vi "Compute n x n Kernel (SGL).vi"(9 "Kernel Type":T1, 11 "Kernel Size":i32) -> (3 "Kernel":sgl[][](array[numeric]))   [LabVIEW 2021, in "Arrays.lvlib"]
uses:
  Arrays.lvlib
  Kernel Type.ctl
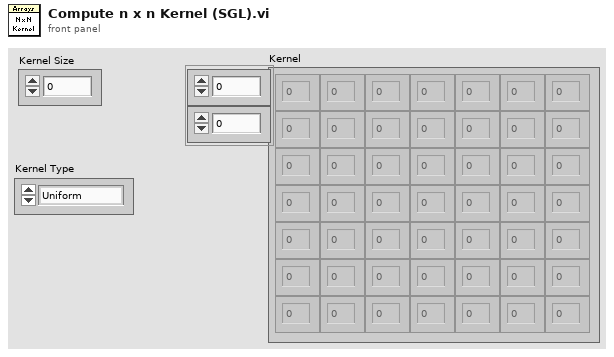
[diagram p1: front panel]
types:
  T1 = typedef "Arrays.lvlib/Kernel Type.ctl" = enum16{"Uniform", "Bilinear", "Gaussian"}
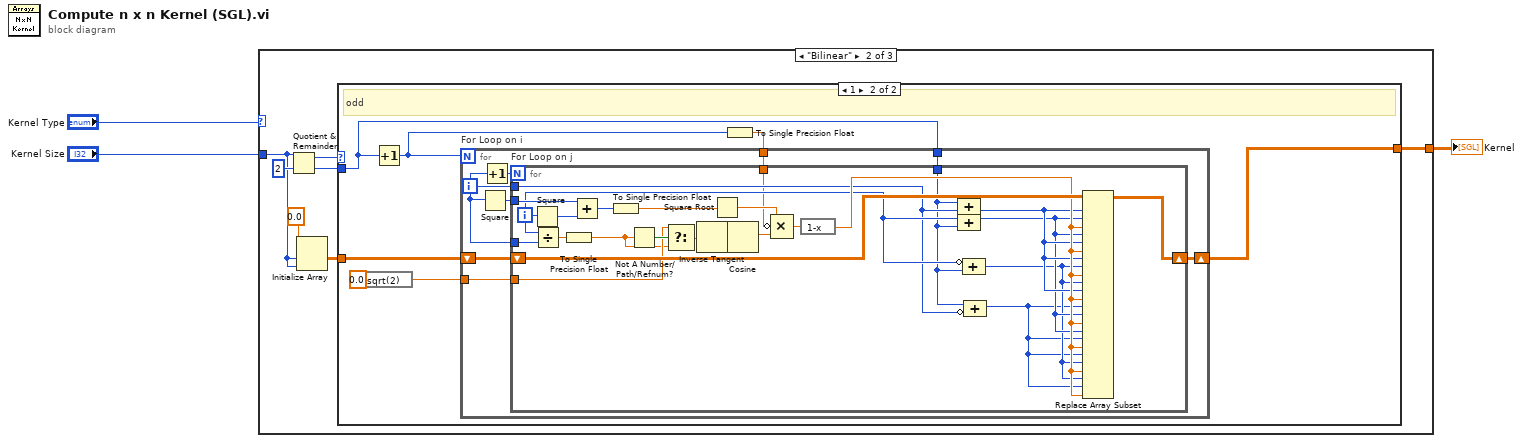
[diagram p0: block diagram]
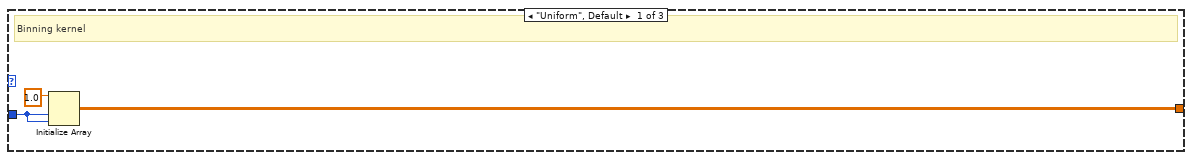
[diagram p2: hidden frame]
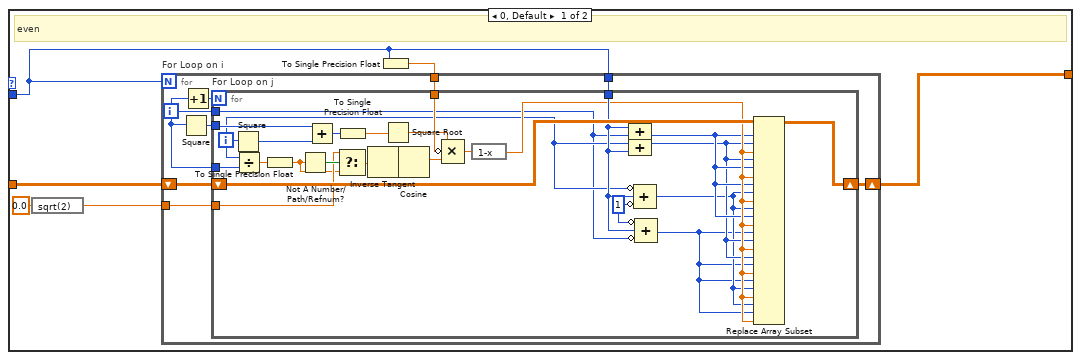
[diagram p3: hidden frame]
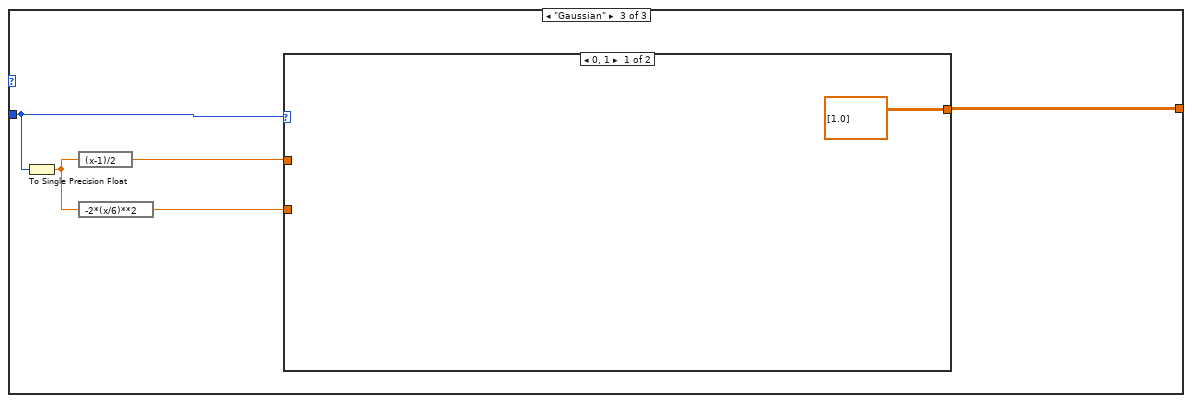
[diagram p4: hidden frame]
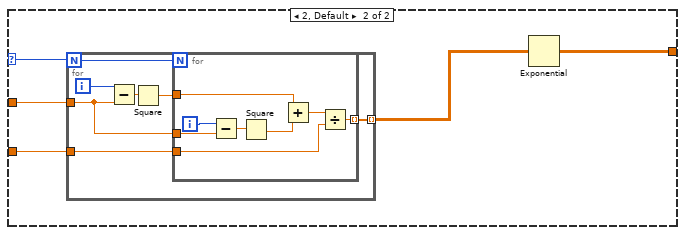
[diagram p5: hidden frame]
diagram:
  n1 = case shown="\"Bilinear\"" "Kernel Type" {
    tunnel: "Kernel Size" -> [w5 w9 w96]
    tunnel: [w4 w7 w98] -> w1
    frame "Uniform", Default {
      # "Binning kernel"
      n2 = Initialize Array(sgl 1.0 ("element"), w5, w5) -> (w4:sgl[][])
    }
    frame "Bilinear" {
      n3 = Quotient & Remainder(x=w9, y=2) -> (x-y*floor(x/y)=w12:i32, floor(x/y)=w11:i32)
      n4 = Initialize Array(sgl 0.0 ("element"), w9, w9) -> (w8:sgl[][])
      n5 = case shown="1" w12 {
        tunnel: w11 -> [w15 w56]
        tunnel: w8 -> [w19 w60]
        tunnel: [w18 w59] -> w7
        frame 0, Default {
          # "even"
          n6 = expression code="sqrt(2)"(sgl 0.0) -> (w17:sgl)
          n7 = To Single Precision Float(number=w15) -> (single precision float=w14:sgl)
          n8 = for "For Loop on i" {
            N: w15 -> [_]
            shift-right: [w25] -> w18
            shift-left: w19 -> [w26]
            tunnel: w14 -> [w23]
            tunnel: w15 -> [w21]
            tunnel: w17 -> [w20]
            i -> [w22]
            n9 = Square(x=w22) -> (x^2=w24:i32)
            n10 = Increment(x=w22) -> (x+1=w27:i32)
            n11 = for "For Loop on j" {
              N: w27 -> [_]
              shift-right: [w43] -> w25
              shift-left: w26 -> [w44]
              tunnel: w24 -> [w52]
              tunnel: w22 -> [w50]
              tunnel: w23 -> [w47]
              tunnel: w22 -> [w31]
              tunnel: w21 -> [w42]
              tunnel: w20 -> [w38]
              i -> [w32]
              w30 = 1 ("value")
              n12 = Square(x=w32) -> (x^2=w53:i32)
              n13 = Divide(x=w32, y=w50) -> (x/y=w37:dbl)
              n14 = To Single Precision Float(number=w37) -> (single precision float=w29:sgl)
              n15 = Not A Number/Path/Refnum?(number/path/refnum=w29) -> (NaN/Path/Refnum?=w40:bool)
              n16 = Add(x=w52, y=w53) -> (x+y=w51:i32)
              n17 = Select(t=w38, s=w40, f=w29) -> (s? t:f=w39:sgl)
              n18 = To Single Precision Float(number=w51) -> (single precision float=w28:sgl)
              n19 = Inverse Tangent(1:w39) -> (0:w49:sgl)
              n20 = Square Root(x=w28) -> (sqrt(x)=w46:sgl)
              n21 = Cosine(x=w49) -> (cos(x)=w48:sgl)
              n22 = Compound Arithmetic op=MULTIPLY(w46, invert w47, w48) -> (w45:sgl)
              n23 = expression code="1-x"(w45) -> (w41:sgl)
              n24 = Compound Arithmetic op=unknown(w42, w31) -> (w36:i32)
              n25 = Compound Arithmetic op=ADD(w32, w42) -> (w35:i32)
              n26 = Compound Arithmetic op=ADD(invert w32, w42, invert w30) -> (w34:i32)
              n27 = Compound Arithmetic op=unknown(invert w30, w42, invert w31) -> (w33:i32)
              n28 = Replace Array Subset(array=w44, new element #1=w41, index (row) #1=w36, index (col) #1=w35, new element #2=w41, index (row) #2=w35, index (col) #2=w36, new element #3=w41, index (row) #3=w36, index (col) #3=w34, new element #4=w41, index (row) #4=w34, index (col) #4=w36, new element #5=w41, index (row) #5=w33, index (col) #5=w35, new element #6=w41, index (row) #6=w35, index (col) #6=w33, new element #7=w41, index (row) #7=w33, index (col) #7=w34, new element #8=w41, index (row) #8=w34, index (col) #8=w33) -> (w43:sgl[][])
            }
          }
        }
        frame 1 {
          # "odd"
          n29 = expression code="sqrt(2)"(sgl 0.0) -> (w58:sgl)
          n30 = Increment(x=w56) -> (x+1=w55:i32)
          n31 = To Single Precision Float(number=w55) -> (single precision float=w54:sgl)
          n32 = for "For Loop on i" {
            N: w55 -> [_]
            shift-right: [w66] -> w59
            shift-left: w60 -> [w67]
            tunnel: w54 -> [w64]
            tunnel: w58 -> [w62]
            tunnel: w56 -> [w61]
            i -> [w63]
            n33 = Square(x=w63) -> (x^2=w65:i32)
            n34 = Increment(x=w63) -> (x+1=w68:i32)
            n35 = for "For Loop on j" {
              N: w68 -> [_]
              shift-right: [w84] -> w66
              shift-left: w67 -> [w85]
              tunnel: w65 -> [w92]
              tunnel: w63 -> [w90]
              tunnel: w64 -> [w72]
              tunnel: w63 -> [w73]
              tunnel: w62 -> [w80]
              tunnel: w61 -> [w71]
              i -> [w74]
              n36 = Square(x=w74) -> (x^2=w93:i32)
              n37 = Divide(x=w74, y=w90) -> (x/y=w79:dbl)
              n38 = To Single Precision Float(number=w79) -> (single precision float=w70:sgl)
              n39 = Add(x=w92, y=w93) -> (x+y=w91:i32)
              n40 = To Single Precision Float(number=w91) -> (single precision float=w69:sgl)
              n41 = Not A Number/Path/Refnum?(number/path/refnum=w70) -> (NaN/Path/Refnum?=w82:bool)
              n42 = Select(t=w80, s=w82, f=w70) -> (s? t:f=w81:sgl)
              n43 = Inverse Tangent(1:w81) -> (0:w89:sgl)
              n44 = Square Root(x=w69) -> (sqrt(x)=w87:sgl)
              n45 = Cosine(x=w89) -> (cos(x)=w88:sgl)
              n46 = Compound Arithmetic op=MULTIPLY(w87, invert w72, w88) -> (w86:sgl)
              n47 = expression code="1-x"(w86) -> (w83:sgl)
              n48 = Compound Arithmetic op=unknown(w71, w73) -> (w78:i32)
              n49 = Compound Arithmetic op=ADD(w74, w71) -> (w77:i32)
              n50 = Compound Arithmetic op=ADD(invert w74, w71) -> (w76:i32)
              n51 = Compound Arithmetic op=unknown(w71, invert w73) -> (w75:i32)
              n52 = Replace Array Subset(array=w85, new element #1=w83, index (row) #1=w78, index (col) #1=w77, new element #2=w83, index (row) #2=w77, index (col) #2=w78, new element #3=w83, index (row) #3=w78, index (col) #3=w76, new element #4=w83, index (row) #4=w76, index (col) #4=w78, new element #5=w83, index (row) #5=w75, index (col) #5=w77, new element #6=w83, index (row) #6=w77, index (col) #6=w75, new element #7=w83, index (row) #7=w75, index (col) #7=w76, new element #8=w83, index (row) #8=w76, index (col) #8=w75) -> (w84:sgl[][])
            }
          }
        }
      }
    }
    frame "Gaussian" {
      n53 = To Single Precision Float(number=w96) -> (single precision float=w97:sgl)
      n54 = expression code="(x-1)/2"(w97) -> (w95:sgl)
      n55 = expression code="-2*(x/6)**2"(w97) -> (w94:sgl)
      n56 = case shown="0, 1" w96 {
        selector: w96 -> [_ w104]
        tunnel: [sgl[][] [[1.0]] w100] -> w98
        tunnel: w95 -> [_ w103]
        tunnel: w94 -> [_ w102]
        frame 0, 1 {
        }
        frame 2, Default {
          n57 = for {
            N: w104 -> [w111]
            tunnel: w103 -> [w108]
            tunnel: w102 -> [w106]
            tunnel: [w105] -> w101 mode=indexing
            i -> [w110]
            n58 = Subtract(x=w110, y=w108) -> (x-y=w109:sgl)
            n59 = Square(x=w109) -> (x^2=w107:sgl)
            n60 = for {
              N: w111 -> [_]
              tunnel: w107 -> [w116]
              tunnel: w108 -> [w118]
              tunnel: w106 -> [w113]
              tunnel: [w112] -> w105 mode=indexing
              i -> [w119]
              n61 = Subtract(x=w119, y=w118) -> (x-y=w117:sgl)
              n62 = Square(x=w117) -> (x^2=w115:sgl)
              n63 = Add(x=w116, y=w115) -> (x+y=w114:sgl)
              n64 = Divide(x=w114, y=w113) -> (x/y=w112:sgl)
            }
          }
          n65 = Exponential(1:w101) -> (0:w100:sgl[][])
        }
      }
    }
  }
  "Kernel" <- w1
